vi "Flush Event.vi"(8 "error in (no error)":errorcluster, 11 "EventMgr in":refnum<class "EventMgr.lvclass">) -> (0 "error out":errorcluster, 1 "Events Remaining":i32, 2 "Event Flushed":refnum<class "Event.lvclass">, 3 "EventMgr out":refnum<class "EventMgr.lvclass">)   [LabVIEW 2013, in "EventMgr.lvclass"]
uses:
  EventMgr.lvclass
  Utilities/Event/Event.lvclass
  EventMgr.lvclass/EventMgr.ctl
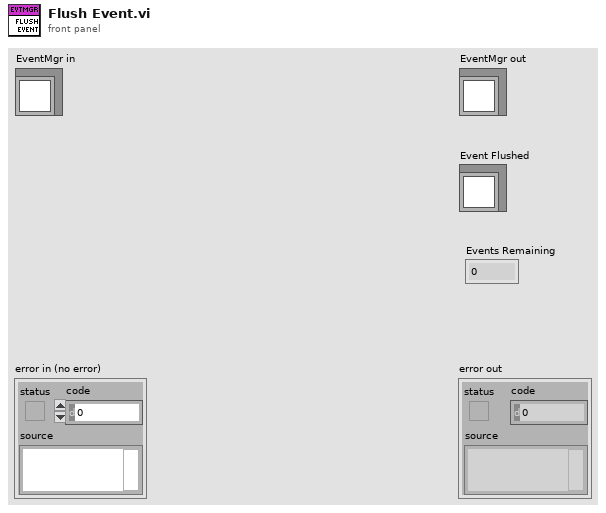
[diagram p1: front panel]
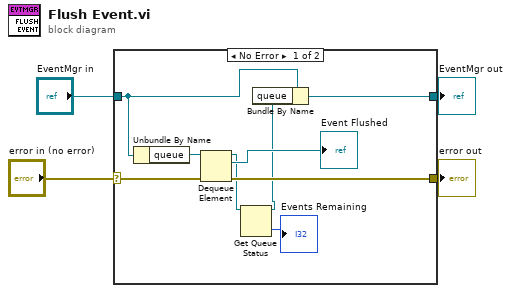
[diagram p0: block diagram]
diagram:
  n1 = case shown="No Error" "error in (no error)" {
    selector: "error in (no error)" -> [w9 w15]
    tunnel: [w8 w15] -> w3
    tunnel: [w11 w14] -> w1
    tunnel: "EventMgr in" -> [w13 w14]
    frame No Error {
      n2 = Unbundle By Name(w13) -> ("queue"=w12:refnum<queue>)
      n3 = Dequeue Element(queue=w12, error in (no error)=w9) -> (queue out=w7:refnum<queue>, element=→"Event Flushed":refnum<class "Event.lvclass">, error out=w8:errorcluster)  [unwired: 1 in, 1 out]
      n4 = Get Queue Status(queue=w7) -> (queue out=w6:refnum<queue>, # elements in queue=→"Events Remaining":i32)  [unwired: 2 in, 6 out]
      n5 = Bundle By Name(cluster=w13, "queue"=w6) -> (w11:refnum<class "EventMgr.lvclass">)
    }
    frame Error {
    }
  }
  "error out" <- w3
  "EventMgr out" <- w1
